vi "Bluetooth_control.vi"() -> ()   [LabVIEW 2016]
uses:
  <vilib>/NXT/NXT Controls/ConnectionType.ctl
  <vilib>/NXT/Block Support/NXT_OutputPort.ctl
  <vilib>/Utility/inputDevices.llb/keyboardAcquire.vi
  <vilib>/NXT/NXTIO Xnodes/NXTIONodeSubVIs/NXTStopMotors.vi
  <vilib>/NXT/NXTIO Xnodes/NXTIONodeSubVIs/NXTMoveMotors.vi
  <vilib>/Utility/inputDevices.llb/closeKeyboard.vi
  <vilib>/NXT/NXTIO Xnodes/AddressXNode/NXTIOAddress.xnode
  <vilib>/NXT/NXTIO Xnodes/NXTIOXNode/NXTIO.xnode
  <vilib>/NXT/Subs/LVHSConnector.ctl
  <vilib>/NXT/LegoClasses/BrickReference/BrickReference.lvclass
panel:
  in  "stop":bool
  out "keys pressed":T1(array[ring])
  # "Indikátor"
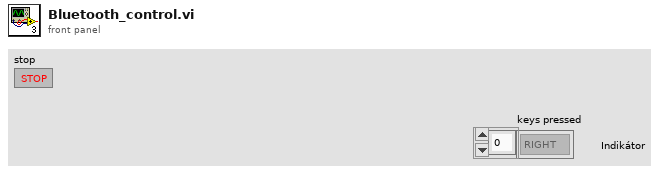
[diagram p1: front panel]
types:
  T1 = enum16{"0", "1", "2", "3", "4", "5", "6", "7", "8", "9", "A", "B", "C", "D", "E", "F", "G", "H", "I", "J", "K", "L", "M", "N", "O", "P", "Q", "R", "S", "T", "U", "V", "W", "X", "Y", "Z", "F1", "F2", "F3", "F4", "F5", "F6", "F7", "F8", "F9", "F10", "F11", "F12", "F13", "F14", "F15", "ADD", "BACK", "BACKSLASH", "CAPITAL", "COMMA", "DECIMAL", "DELETE", "DIVIDE", "DOWN", "END", "EQUALS", "ESCAPE", "GRAVE (`)", "HOME", "INSERT", "LBRACKET", "LCONTROL", "LEFT", "L ALT", "LSHIFT", "LWIN", "MINUS", "MULTIPLY", "NEXT", "NUMLOCK", "NUMPAD_0", "NUMPAD_1", "NUMPAD_2", "NUMPAD_3", "NUMPAD_4", "NUMPAD_5", "NUMPAD_6", "NUMPAD_7", "NUMPAD_8", "NUMPAD_9", "PAUSE", "PERIOD", "PRIOR (PG UP)", "RBRACKET", "RCONTROL", "RETURN", "RIGHT", "R ALT", "RSHIFT", "RWIN", "SCROLL", "SEMICOLON", "SLASH", "SPACE", "SUBTRACT", "TAB", "UP", "ENTER (num pad)", "' (quote)"}[]
  T2 = typedef "ConnectionType.ctl" = enum16{"Bluetooth", "USB", "WiFi"}
  T3 = typedef "LVHSConnector.ctl" = refnum<class "BrickReference.lvclass">
  T4 = typedef "NXT_OutputPort.ctl" = u8
  T5 = enum16{"0", "1", "2", "3", "4", "5", "6", "7", "8", "9", "A", "B", "C", "D", "E", "F", "G", "H", "I", "J", "K", "L", "M", "N", "O", "P", "Q", "R", "S", "T", "U", "V", "W", "X", "Y", "Z", "F1", "F2", "F3", "F4", "F5", "F6", "F7", "F8", "F9", "F10", "F11", "F12", "F13", "F14", "F15", "ADD", "BACK", "BACKSLASH", "CAPITAL", "COMMA", "DECIMAL", "DELETE", "DIVIDE", "DOWN", "END", "EQUALS", "ESCAPE", "GRAVE (`)", "HOME", "INSERT", "LBRACKET", "LCONTROL", "LEFT", "L ALT", "LSHIFT", "LWIN", "MINUS", "MULTIPLY", "NEXT", "NUMLOCK", "NUMPAD_0", "NUMPAD_1", "NUMPAD_2", "NUMPAD_3", "NUMPAD_4", "NUMPAD_5", "NUMPAD_6", "NUMPAD_7", "NUMPAD_8", "NUMPAD_9", "PAUSE", "PERIOD", "PRIOR (PG UP)", "RBRACKET", "RCONTROL", "RETURN", "RIGHT", "R ALT", "RSHIFT", "RWIN", "SCROLL", "SEMICOLON", "SLASH", "SPACE", "SUBTRACT", "TAB", "UP", "ENTER (num pad)", "' (quote)"}
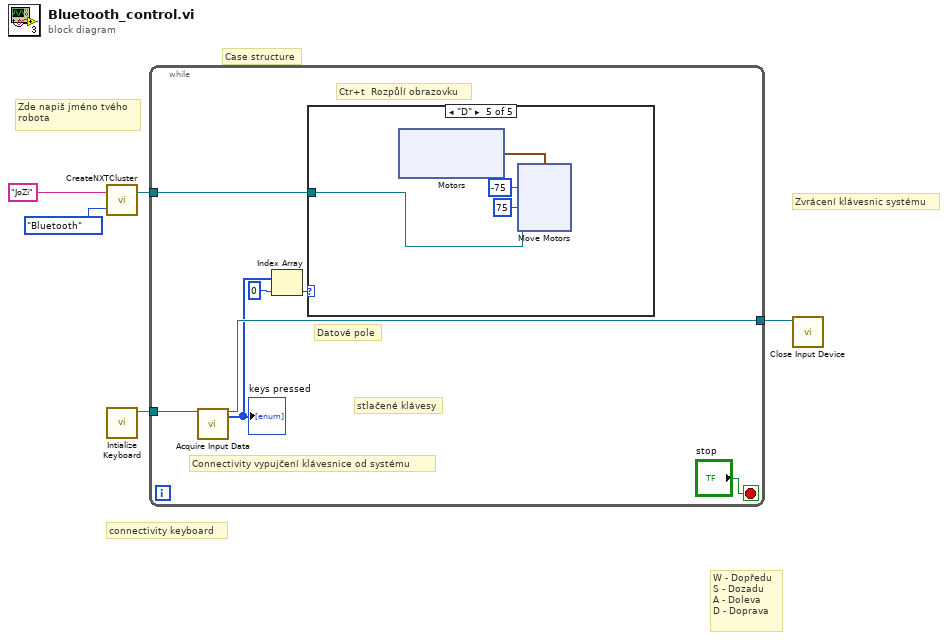
[diagram p0: block diagram]
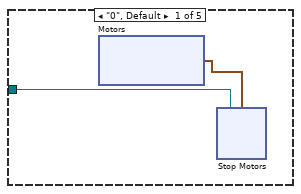
[diagram p2: hidden frame]
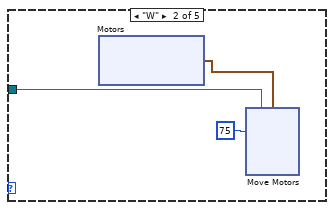
[diagram p3: hidden frame]
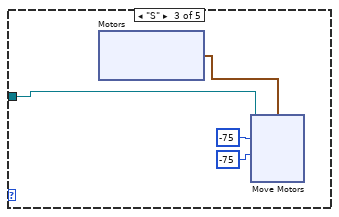
[diagram p4: hidden frame]
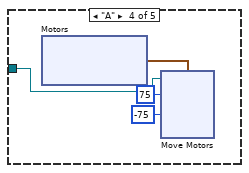
[diagram p5: hidden frame]
diagram:
  # "Zde napiš jméno tvého\nrobota"
  # "W - Dopředu\nS - Dozadu\nA - Doleva\nD - Doprava"
  # "Case structure"
  # "Zvrácení klávesnic systému"
  # "connectivity keyboard"
  # "Ctr+t  Rozpůlí obrazovku"
  n1 = call <vilib>:"CreateNXTCluster.vi"("Connection Type"=ConnectionType."Bluetooth", "NXT/EV3 name"="JoZi") -> ("NXT/EV3"=w1:T3)  [unwired: 2 in]
  n2 = call <vilib>:"Intialize Keyboard.vi"() -> ("device ID"=w5:refnum<k1>)  [unwired: 10 in, 1 out]
  n3 = while {
    tunnel: w5 -> [w12]
    tunnel: [w11] -> w4
    tunnel: w1 -> [w6]
    stop <- "stop" stop-if-true
    # "stlačené klávesy"
    # "Datové pole"
    # "Connectivity vypujčení klávesnice od systému"
    n4 = call-poly <vilib>:"Acquire Input Data.vi"("device ID"=w12) -> ("device ID"=w11:refnum<k1>, "keys pressed"=w9:T1)  [unwired: 16 in, 1 out]
    "keys pressed" <- w9
    n5 = Index Array(array=w9, index=0) -> (element=w7:T5)
    n6 = case shown="\"D\"" w7 {
      tunnel: w6 -> [w13 w22 w33 w48 w59]
      frame "0", Default {
        n7 = xnode "Motors"() -> ("Motor"=w14:cluster{"Port":T4, "Port":T4})
        n8 = xnode "Stop Motors"("Motors"=w14, "NXT/EV3"=w13) -> ()  [unwired: 1 out]
      }
      frame "W" {
        n9 = xnode "Motors"() -> ("Motor"=w21:cluster{"Port":T4, "Port":T4})
        n10 = xnode "Move Motors"("Power/Speed 1"=i8 75, "Motors"=w21, "NXT/EV3"=w22) -> ()  [unwired: 1 in, 1 out]
      }
      frame "S" {
        n11 = xnode "Motors"() -> ("Motor"=w35:cluster{"Port":T4, "Port":T4})
        n12 = xnode "Move Motors"("Power/Speed 2"=i8 -75, "Power/Speed 1"=i8 -75, "Motors"=w35, "NXT/EV3"=w33) -> ()  [unwired: 1 out]
      }
      frame "A" {
        n13 = xnode "Motors"() -> ("Motor"=w49:cluster{"Port":T4, "Port":T4})
        n14 = xnode "Move Motors"("Power/Speed 2"=i8 -75, "Power/Speed 1"=i8 75, "Motors"=w49, "NXT/EV3"=w48) -> ()  [unwired: 1 out]
      }
      frame "D" {
        n15 = xnode "Motors"() -> ("Motor"=w62:cluster{"Port":T4, "Port":T4})
        n16 = xnode "Move Motors"("Power/Speed 2"=i8 75, "Power/Speed 1"=i8 -75, "Motors"=w62, "NXT/EV3"=w59) -> ()  [unwired: 1 out]
      }
    }
  }
  n17 = call-poly <vilib>:"Close Input Device.vi"("device ID"=w4) -> ()  [unwired: 9 in, 1 out]
